vi "Pulse Timer Test Bench.vi"() -> ()   [LabVIEW 2014]
panel:
  out "Pulse Out":bool
  in  "On Time":u32=1
  in  "Off Time":u32=20
  in  "Pulse State":bool
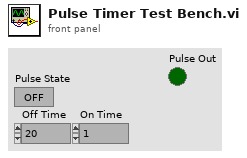
[diagram p1: front panel]
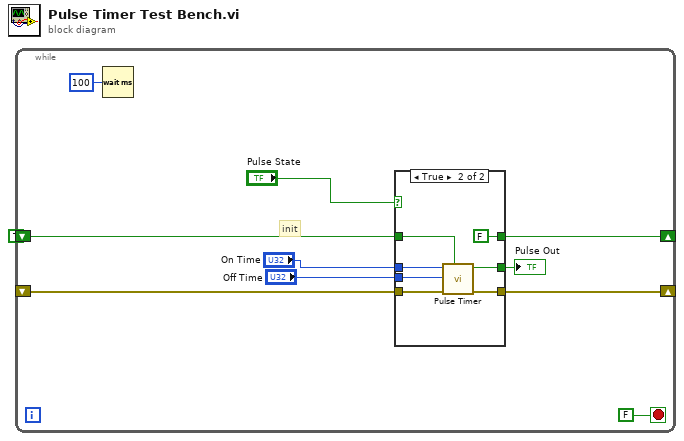
[diagram p0: block diagram]
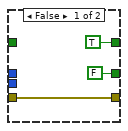
[diagram p2: hidden frame]
diagram:
  n1 = while {
    shift-right: [w8] -> _
    shift-left: _ -> [w7]
    shift-right: [w3] -> _
    shift-left: TRUE ("Boolean Out") -> [w2]
    stop <- FALSE stop-if-true
    # "init"
    n2 = Wait (ms)(milliseconds to wait=u32 100) -> ()  [unwired: 1 out]
    n3 = case shown="True" "Pulse State" {
      tunnel: [w12 w21] -> w8
      tunnel: w7 -> [w12 w20]
      tunnel: "Off Time" -> [_ w19]
      tunnel: "On Time" -> [_ w18]
      tunnel: [FALSE ("Boolean Out") w17] -> w4
      tunnel: [TRUE ("Boolean Out") FALSE ("Boolean Out")] -> w3
      tunnel: w2 -> [_ w16]
      frame False {
      }
      frame True {
        n4 = call "Pulse Timer.vi"("Initialize"=w16, "Error In"=w20, "Off Time"=w19, "On Time"=w18) -> ("Error Out"=w21:errorcluster, "Boolean Out"=w17:bool)  [unwired: 6 in]
      }
    }
    "Pulse Out" <- w4
  }
